vi "waveform test.vi"() -> ()   [LabVIEW 2013]
uses:
  Libraries/California Instruments iX Series/California Instruments iX Series.lvlib
panel:
  out "Waveform Graph 2":sgl[](graph)
  out "return count 2":u32
  out "Numeric 2":i32
  out "Serial Settings:Number \nof Bytes at Serial Port 2":u32
  out "Waveform Graph":sgl[](graph)
  out "Numeric":i32
  out "error out":errorcluster
  in  "Multiple Voltage Measurement Type (0:DC)":u16(ring) items=["Voltage", "Voltage Harmonic Amplitude", "Voltage Harmonic Phase"]
  out "Voltage Measurements":sgl[](array[numeric])
  out "return count":u32
  out "Serial Settings:Number \nof Bytes at Serial Port":u32
  out "size(s)":i32
  in  "error in (no error)":errorcluster
  in  "VISA resource name":refnum<visa-resource-name>
  in  "Serial Configuration":cluster{"Baud Rate":u32, "Flow Control":u16}={"Baud Rate"=460800, "Flow Control"=0} {"Flow Control" items=["None", "XON/XOFF", "RTS/CTS", "XON/XOFF & RTS/CTS", "DTR/DSR", "XON/XOFF & DTR/DSR"]; "Baud Rate" items=["9600"=9600, "19200"=19200, "38400"=38400, "57600"=57600, "115200"=115200, "230400"=230400, "460800"=460800]}
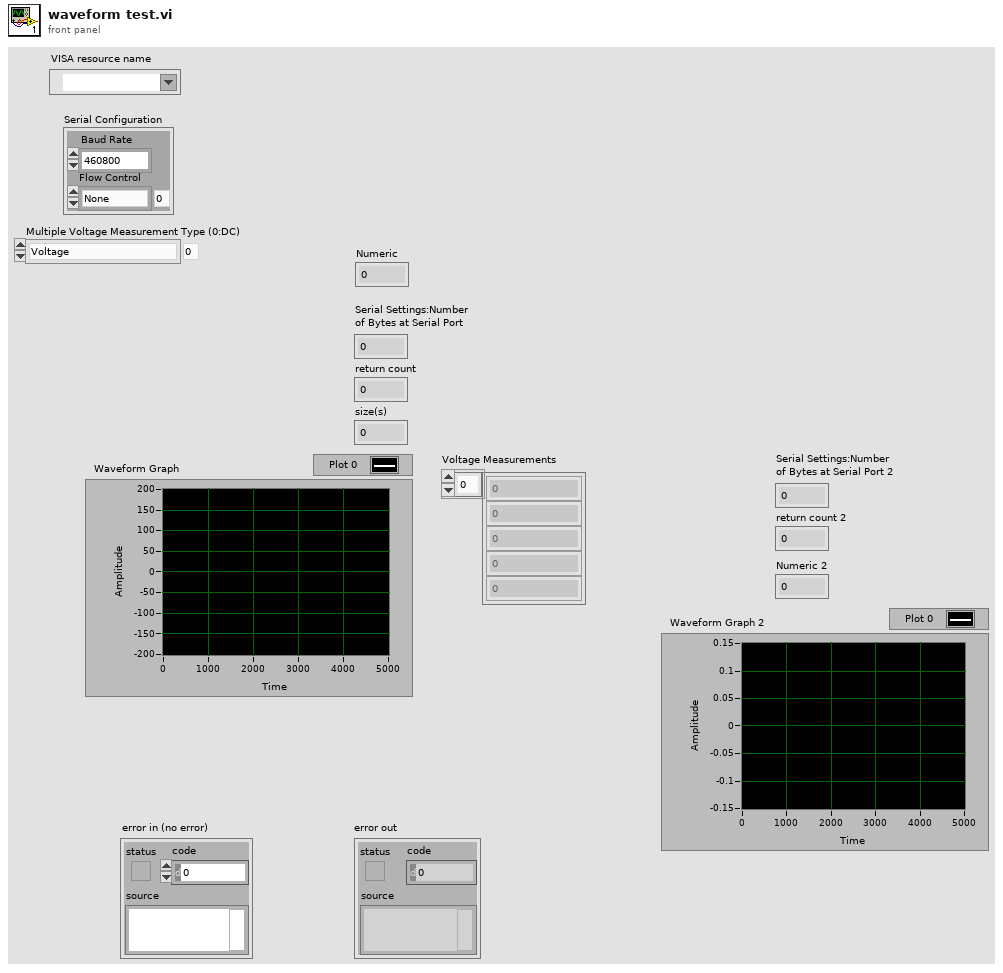
[diagram p1: front panel]
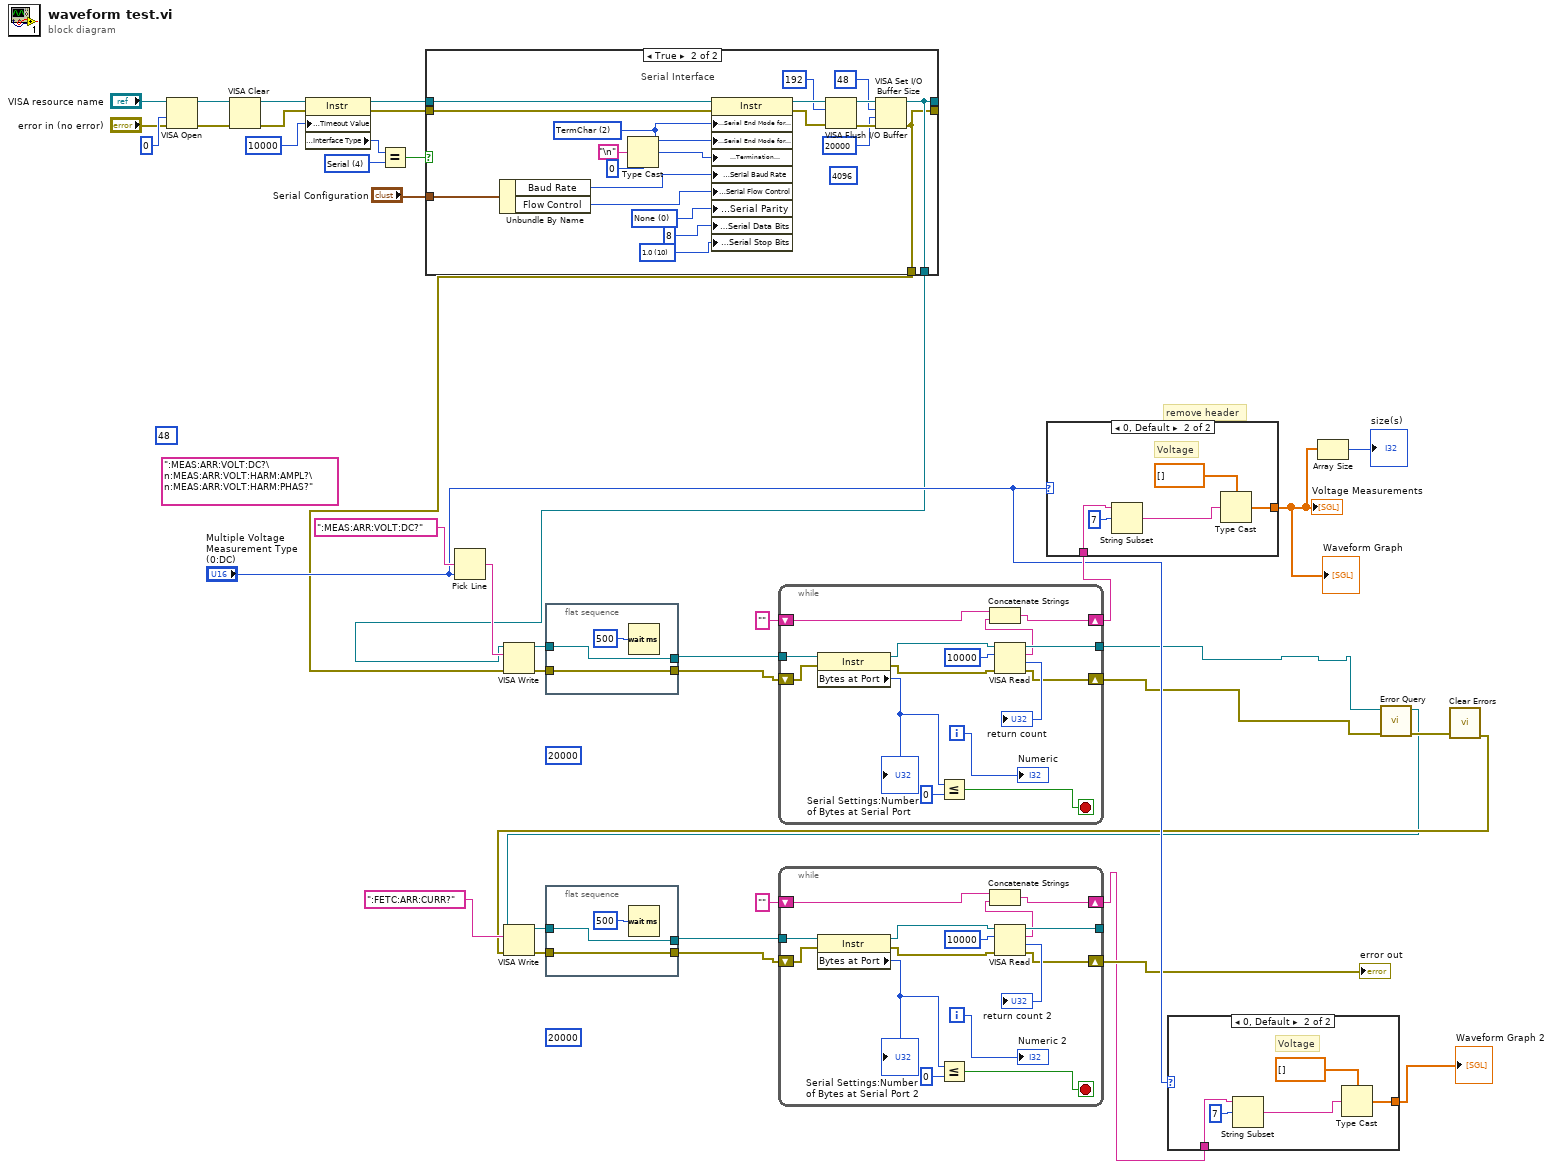
[diagram p0: block diagram]
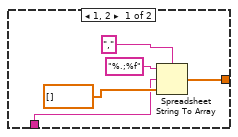
[diagram p2: hidden frame]
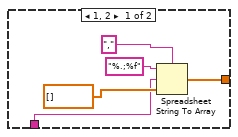
[diagram p3: hidden frame]
diagram:
  (unwired) u32 20000 ("size (4096)")
  (unwired) u16 48 ("mask (16)")
  (unwired) u32 20000 ("size (4096)")
  (unwired) ":MEAS:ARR:VOLT:DC?\n:MEAS:ARR:VOLT:HARM:AMPL?\n:MEAS:ARR:VOLT:HARM:PHAS?" ("multi-line string")
  w35 = u16 4 items=["GPIB"=1, "VXI"=2, "GPIB-VXI"=3, "Serial"=4, "PXI"=5, "TCPIP"=6, "USB"=7] ("Interface Information:Interface Type")
  # "remove header"
  n1 = VISA Open(access mode=u32 0, error in (no error)="error in (no error)", VISA resource name="VISA resource name") -> (VISA resource name=w37:refnum<visa-resource-name>, error out=w38:errorcluster)  [unwired: 2 in]
  n2 = VISA Clear(VISA resource name=w37, error in (no error)=w38) -> (VISA resource name out=w39:refnum<visa-resource-name>, error out=w40:errorcluster)
  n3 = property class="Instr"(reference=w39, error in=w40, "General Settings:Timeout Value"=u32 10000) -> (reference out=w32:refnum<visa-resource-name>, error out=w33:errorcluster, "Interface Information:Interface Type"=w30:u16)
  n4 = Equal?(x=w30, y=w35) -> (x = y?=w34:bool)
  n5 = case shown="True" w34 {
    tunnel: [w42 w46] -> _
    tunnel: [w43 w45] -> _
    tunnel: w32 -> [w42 w63]
    tunnel: w33 -> [w43 w64]
    tunnel: "Serial Configuration" -> [_ w51]
    tunnel: [_ w46] -> w2
    tunnel: [_ w45] -> w1
    frame False {
      # "GPIB, TCP/IP, and USB Interface"
    }
    frame True {
      (unwired) u32 4096 ("size (0)")
      w48 = u16 0 items=["None", "Odd", "Even", "Mark", "Space"] ("Serial Settings:Parity")
      w50 = u16 10 items=["1.0"=10, "1.5"=15, "2.0"=20] ("Serial Settings:Stop Bits")
      w55 = u16 2 items=["None", "LastBit", "TermChar"] ("Serial Settings:Serial End Mode for Reads")
      # "Serial Interface"
      n6 = Unbundle By Name(w51) -> ("Baud Rate"=w53:u32, "Flow Control"=w52:u16)
      n7 = Type Cast(type=u8 0, x="\n" ("Line Feed Constant")) -> (*(type *) &x=w54:u8)
      n8 = property class="Instr"(reference=w63, error in=w64, "Serial Settings:Serial End Mode for Reads"=w55, "Serial Settings:Serial End Mode for Writes"=w55, "Message Based Settings:Termination Character"=w54, "Serial Settings:Serial Baud Rate"=w53, "Serial Settings:Serial Flow Control"=w52, "Serial Settings:Serial Parity"=w48, "Serial Settings:Serial Data Bits"=u16 8 ("Serial Settings:Data Bits"), "Serial Settings:Serial Stop Bits"=w50) -> (reference out=w59:refnum<visa-resource-name>, error out=w61:errorcluster)
      n9 = VISA Flush I/O Buffer(VISA resource name=w59, mask (16)=u16 192, error in (no error)=w61) -> (VISA resource name out=w62:refnum<visa-resource-name>, error out=w60:errorcluster)
      n10 = VISA Set I/O Buffer Size(VISA resource name=w62, mask (16)=u16 48, size (4096)=u32 20000 ("size (0)"), error in (no error)=w60) -> (VISA resource name out=w46:refnum<visa-resource-name>, error out=w45:errorcluster)
    }
  }
  n11 = Pick Line(multi-line string=":MEAS:ARR:VOLT:DC?", line index="Multiple Voltage Measurement Type (0:DC)") -> (output string=w24:string)  [unwired: 1 in]
  n12 = VISA Write(VISA resource name=w2, write buffer=w24, error in (no error)=w1) -> (VISA resource name out=w25:refnum<visa-resource-name>, error out=w26:errorcluster)  [unwired: 1 out]
  n13 = flat-sequence {
    tunnel: w25 -> [w66]
    tunnel: [w66] -> w22
    tunnel: w26 -> [w65]
    tunnel: [w65] -> w21
    frame #0 {
      n14 = Wait (ms)(milliseconds to wait=u32 500) -> ()  [unwired: 1 out]
    }
  }
  n15 = flat-sequence {
    tunnel: w10 -> [w69]
    tunnel: [w69] -> w11
    tunnel: w9 -> [w68]
    tunnel: [w68] -> w12
    frame #0 {
      n16 = Wait (ms)(milliseconds to wait=u32 500) -> ()  [unwired: 1 out]
    }
  }
  n17 = while {
    tunnel: [w84] -> w16
    shift-right: [w71] -> w20
    shift-left: "" -> [w82]
    tunnel: w22 -> [w79]
    shift-right: [w75] -> w15
    shift-left: w21 -> [w76]
    i -> [w80]
    stop <- w72 stop-if-true
    n18 = property class="Instr"(reference=w79, error in=w76) -> (reference out=w78:refnum<visa-resource-name>, error out=w77:errorcluster, "Bytes at Port"=w74:u32)
    "Serial Settings:Number \nof Bytes at Serial Port" <- w74
    n19 = Less Or Equal?(x=w74, y=u32 0) -> (x <= y?=w72:bool)
    n20 = VISA Read(VISA resource name=w78, byte count=u32 10000, error in (no error)=w77) -> (VISA resource name out=w84:refnum<visa-resource-name>, read buffer=w81:string, return count=→"return count":u32, error out=w75:errorcluster)
    n21 = Concatenate Strings(w82, w81) -> (w71:string)
    "Numeric" <- w80
  }
  n22 = while {
    tunnel: [w99] -> _
    shift-right: [w86] -> w6
    shift-left: "" -> [w97]
    tunnel: w11 -> [w94]
    shift-right: [w90] -> w7
    shift-left: w12 -> [w91]
    i -> [w95]
    stop <- w87 stop-if-true
    n23 = property class="Instr"(reference=w94, error in=w91) -> (reference out=w93:refnum<visa-resource-name>, error out=w92:errorcluster, "Bytes at Port"=w89:u32)
    "Serial Settings:Number \nof Bytes at Serial Port 2" <- w89
    n24 = Less Or Equal?(x=w89, y=u32 0) -> (x <= y?=w87:bool)
    n25 = VISA Read(VISA resource name=w93, byte count=u32 10000, error in (no error)=w92) -> (VISA resource name out=w99:refnum<visa-resource-name>, read buffer=w96:string, return count=→"return count 2":u32, error out=w90:errorcluster)
    n26 = Concatenate Strings(w97, w96) -> (w86:string)
    "Numeric 2" <- w95
  }
  "error out" <- w7
  n27 = case shown="0, Default" "Multiple Voltage Measurement Type (0:DC)" {
    tunnel: [w103 w107] -> w18
    tunnel: w20 -> [w101 w106]
    frame 1, 2 {
      n28 = Spreadsheet String To Array(delimiter (Tab)=",", format string="%.;%f", spreadsheet string=w101, array type (2D Dbl)=sgl[] []) -> (array=w103:sgl[])
    }
    frame 0, Default {
      # "Voltage"
      n29 = String Subset(string=w106, offset (0)=7) -> (substring=w109:string)  [unwired: 1 in]
      n30 = Type Cast(type=sgl[] [], x=w109) -> (*(type *) &x=w107:sgl[])
    }
  }
  "Voltage Measurements" <- w18
  "Waveform Graph" <- w18
  n31 = case shown="0, Default" "Multiple Voltage Measurement Type (0:DC)" {
    tunnel: [w113 w117] -> w5
    tunnel: w6 -> [w111 w116]
    frame 1, 2 {
      n32 = Spreadsheet String To Array(delimiter (Tab)=",", format string="%.;%f", spreadsheet string=w111, array type (2D Dbl)=sgl[] []) -> (array=w113:sgl[])
    }
    frame 0, Default {
      # "Voltage"
      n33 = String Subset(string=w116, offset (0)=7) -> (substring=w119:string)  [unwired: 1 in]
      n34 = Type Cast(type=sgl[] [], x=w119) -> (*(type *) &x=w117:sgl[])
    }
  }
  "Waveform Graph 2" <- w5
  n35 = Array Size(array=w18) -> (size(s)=→"size(s)":i32)
  n36 = call "Error Query.vi"("error in (no error)"=w15, "VISA resource name"=w16) -> ("error out"=w14:errorcluster, "VISA resource name out"=w3:refnum<visa-resource-name>)  [unwired: 6 in, 2 out]
  n37 = call <vilib>:"Clear Errors.vi"("error in (no error)"=w14) -> ("error out"=w4:errorcluster)  [unwired: 6 in]
  n38 = VISA Write(VISA resource name=w3, write buffer=":FETC:ARR:CURR?" ("multi-line string"), error in (no error)=w4) -> (VISA resource name out=w10:refnum<visa-resource-name>, error out=w9:errorcluster)  [unwired: 1 out]
